vi "Test.vi"() -> ()   [LabVIEW 2020]
uses:
  CTI/I2C Address.ctl
  CTI/Error Reporting.ctl
  CTI/ADC Number.ctl
  CTI/I2C Number.ctl
  CTI/GPIO Number.ctl
  3ecabbcd-11d4-4a0f-8cd7-5b8d660a803b.vi
  CTI/Session/Session.lvclass
  CTI/CTI.lvlib
  CTI/VisaComms/VisaComms.lvclass
panel:
  out "error out":errorcluster
  in  "Port":refnum<visa-resource-name>="COM3"
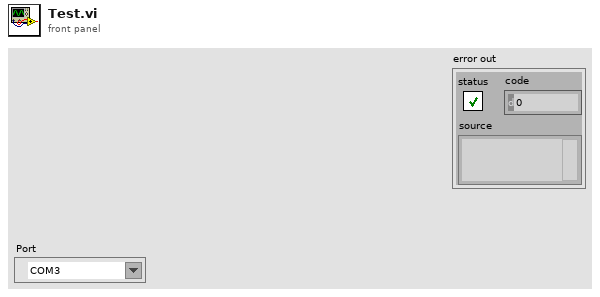
[diagram p1: front panel]
types:
  T1 = typedef "CTI.lvlib/I2C Address.ctl" = u8
  T2 = typedef "CTI.lvlib/Error Reporting.ctl" = enum16{"Minimal", "Moderate", "Full"}
  T3 = typedef "CTI.lvlib/ADC Number.ctl" = i8
  T4 = typedef "CTI.lvlib/GPIO Number.ctl" = i8
  T5 = typedef "CTI.lvlib/I2C Number.ctl" = i8
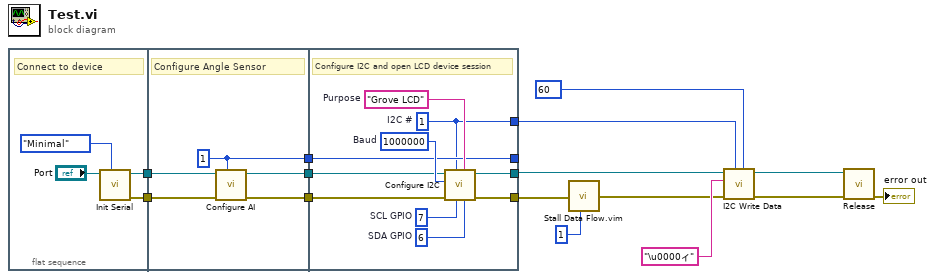
[diagram p0: block diagram]
diagram:
  n1 = flat-sequence {
    tunnel: [w18] -> w15
    tunnel: [w17] -> w14
    tunnel: w15 -> [w23]
    tunnel: w14 -> [w24]
    tunnel: [w22] -> w13
    tunnel: [w21] -> w12
    tunnel: [w20] -> w11
    tunnel: [w27] -> _
    tunnel: w13 -> [w27]
    tunnel: w12 -> [w31]
    tunnel: w11 -> [w29]
    tunnel: [w28] -> w10
    tunnel: [w26] -> w9
    tunnel: [w25] -> w6
    frame #0 {
      # "Connect to device"
      n2 = call "Init Serial.vi"("Error Checking (Full)"=Error_Reporting."Minimal", "VISA resource name in"="Port") -> ("error out"=w17:errorcluster, "Session"=w18:refnum<class "Session.lvclass">)  [unwired: 7 in, 1 out]
    }
    frame #1 {
      w22 = T3 1
      # "Configure Angle Sensor"
      n3 = call "Configure AI.vi"("ADC #"=w22, "error in (no error)"=w24, "Session in"=w23) -> ("error out"=w21:errorcluster, "Session out"=w20:refnum<class "Session.lvclass">)  [unwired: 7 in]
    }
    frame #2 {
      w34 = T4 6  # SDA GPIO
      w32 = T4 7  # SCL GPIO
      w33 = "Grove LCD"  # Purpose
      w25 = T5 1  # I2C #
      w30 = u32 1000000  # Baud
      # "Configure I2C and open LCD device session"
      n4 = call "Configure I2C.vi"("SDA GPIO"=w34, "Purpose (\"I2C\")"=w33, "SCL GPIO"=w32, "I2C #"=w25, "error in (no error)"=w31, "Baud"=w30, "Session in"=w29) -> ("error out"=w26:errorcluster, "Session out"=w28:refnum<class "Session.lvclass">)  [unwired: 3 in]
    }
  }
  n5 = call "Stall Data Flow.vim"("value in"=w9, "milliseconds to wait"=u32 1) -> ("value out"=w2:errorcluster)  [unwired: 1 out]
  n6 = call "I2C Write Data.vi"("Address"=T1 60, "I2C #"=w6, "error in (no error)"=w2, "Data"="\u0000イ", "Session in"=w10) -> ("error out"=w5:errorcluster, "Session out"=w4:refnum<class "Session.lvclass">)  [unwired: 5 in]
  n7 = call-dynamic "Release.vi"("error in (no error)"=w5, "Session in"=w4) -> ("error out"=→"error out":errorcluster)  [unwired: 9 in]
